vi "Utility - Edit Device Tree Items.vi"() -> ()   [LabVIEW 2015]
uses:
  Globals/Global - Device Tree Items - FCXF.vi
panel:
  in  "device tree":string[](tree)=["FCXF-X-03-S05"] caption="设备列表"
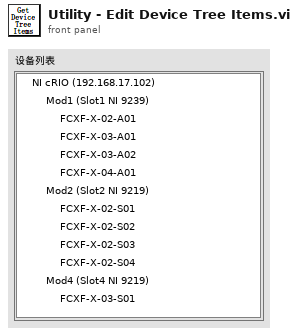
[diagram p1: front panel]
types:
  T1 = cluster{"Left Cell String":string, "Child Text":string[], "Child Tag":string, "Item Indent":i32, "Child Only?":bool, "Glyph Index":i32}
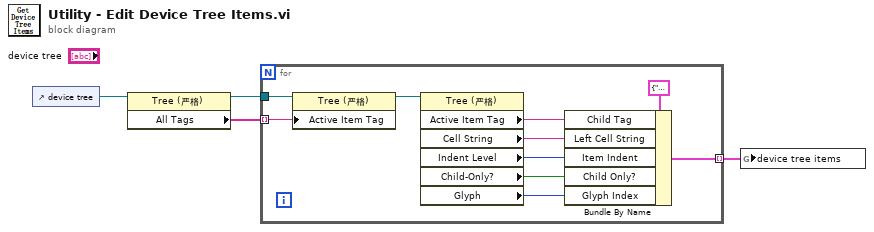
[diagram p0: block diagram]
diagram:
  n1 = control-ref of="device tree"() -> (w4:refnum<vi>)
  n2 = property class="Tree (严格)"(reference=w4) -> (reference out=w3:refnum<vi>, "All Tags"=w2:string[])  [unwired: 1 in, 1 out]
  n3 = for {
    tunnel: w3 -> [w14]
    tunnel: w2 -> [w12] mode=indexing
    tunnel: [w5] -> w1 mode=indexing
    n4 = property class="Tree (严格)"(reference=w14, "Active Item Tag"=w12) -> (reference out=w13:refnum<vi>)  [unwired: 1 in, 1 out]
    n5 = property class="Tree (严格)"(reference=w13) -> ("Active Item Tag"=w10:string, "Cell String"=w9:string, "Indent Level"=w8:i32, "Child-Only?"=w7:bool, "Glyph"=w6:i32)  [unwired: 1 in, 2 out]
    n6 = Bundle By Name(cluster=T1 {"Left Cell String"="FCXF-X-03-T02", "Child Text"=[], "Child Tag"="FCXF-X-03-T02", "Item Indent"=2, "Child Only?"=TRUE, "Glyph Index"=4} ("Item"), "Child Tag"=w10, "Left Cell String"=w9, "Item Indent"=w8, "Child Only?"=w7, "Glyph Index"=w6) -> (w5:T1)
  }
  n7 = global write "Global - Device Tree Items - FCXF.vi" "device tree items"(w1) -> ()
